vi "Add Calculate Channel_Average.vi"(7 "Overwrite Existing?":bool=TRUE, 8 "error in (no error)":errorcluster, 9 "Average Settings":T1={"Name"="", "Description"="", "NumberOfPoints"=10, "Channel Node Path"="", "Alias Name"=""}, 10 "Base Node Path":string, 11 "SysDef Ref":T2) -> (0 "error out":errorcluster, 2 "New Node Path":string, 3 "SysDef Ref Out":T2)   [LabVIEW 2019, in "Simple SysDef API.lvlib"]
uses:
  <userlib>/SimpleSysDef/Simple SysDef API.lvlib
  <userlib>/SimpleSysDef/_SubVIs/System Definition Reference.ctl
  NationalInstruments.VeriStand.SystemDefinitionAPI
  <userlib>/SimpleSysDef/_SubVIs/Add Calculate Channel_Average_Settings.ctl
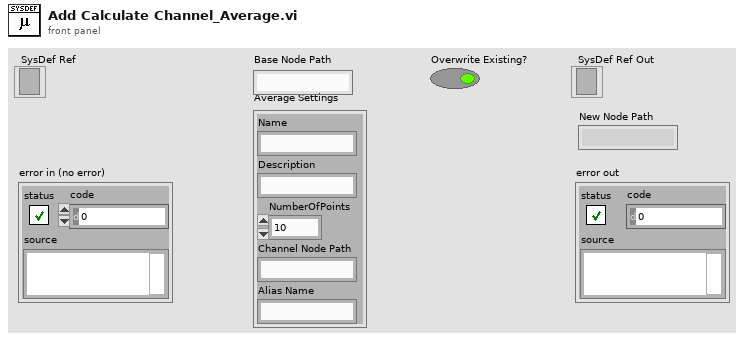
[diagram p1: front panel]
types:
  T1 = typedef "Simple SysDef API.lvlib/Add Calculate Channel_Average_Settings.ctl" = cluster{"Name":string, "Description":string, "NumberOfPoints":u32, "Channel Node Path":string, "Alias Name":string}
  T2 = typedef "Simple SysDef API.lvlib/System Definition Reference.ctl" = refnum<k24>
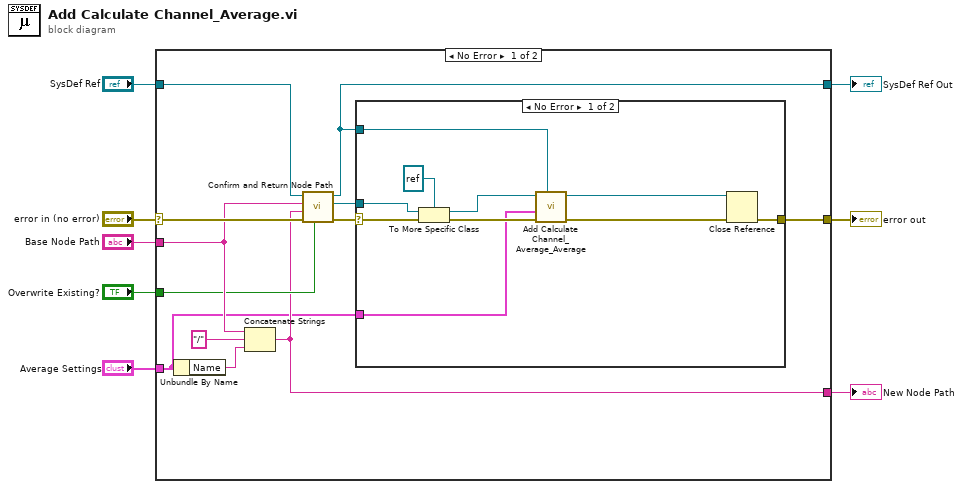
[diagram p0: block diagram]
diagram:
  n1 = case shown="No Error" "error in (no error)" {
    selector: "error in (no error)" -> [w20 w33]
    tunnel: [w16 w33] -> w7
    tunnel: "SysDef Ref" -> [w19 w32]
    tunnel: [w10 w32] -> w5
    tunnel: "Base Node Path" -> [w13 _]
    tunnel: "Overwrite Existing?" -> [w12 _]
    tunnel: "Average Settings" -> [w9 _]
    tunnel: [w11 _] -> w1
    frame No Error {
      n2 = Unbundle By Name(w9) -> ("Name"=w17:string)
      n3 = Concatenate Strings(w13, "/" ("string"), w17) -> (w11:string)
      n4 = call <userlib>:"Confirm and Return Node Path.vi"("Overwrite Existing?"=w12, "error in (no error)"=w20, "New Node Path"=w11, "Base Node Path"=w13, "SysDef Ref"=w19) -> ("error out"=w14:errorcluster, "Node Ref"=w15:refnum<k24>, "SysDef Ref Out"=w10:T2)  [unwired: 4 in]
      n5 = case shown="No Error" w14 {
        selector: w14 -> [w29 w31]
        tunnel: [w28 w31] -> w16
        tunnel: w15 -> [w30 _]
        tunnel: w10 -> [w21 _]
        tunnel: w9 -> [w25 _]
        frame No Error {
          n6 = To More Specific Class(target class=refnum<k24> refnum ("Node Ref"), reference=w30, error in=w29) -> (specific class reference=w24:refnum<k24>, error out=w26:errorcluster)
          n7 = call <userlib>:"Add Calculate Channel_Average_Average.vi"("SysDef Ref"=w21, "error in (error out)"=w26, "Average Settings"=w25, "Calculated Channels Ref"=w24) -> ("error out"=w22:errorcluster, "Calculated Channels Ref Out"=w23:refnum<k24>)  [unwired: 6 in]
          n8 = Close Reference(reference=w23, error in (no error)=w22) -> (error out=w28:errorcluster)
        }
        frame Error {
        }
      }
    }
    frame Error {
    }
  }
  "SysDef Ref Out" <- w5
  "error out" <- w7
  "New Node Path" <- w1
